vi "usrp get rx rates.vi"(8 "error in (no error)":errorcluster, 9 "rates_out":u64, 10 "chan":u64, 11 "h":u64) -> (0 "error out":errorcluster, 3 "function return":u32(ring))   [LabVIEW 2023, in "uhd.lvlib"]
doc: "UHD_API uhd_error uhd_usrp_get_rx_rates(\n uhd_usrp_handle h, size_t chan, uhd_meta_range_handle rates_out);"
uses:
  <userlib>/uhd/uhd.lvlib
  <userlib>/uhd/uhd.dll
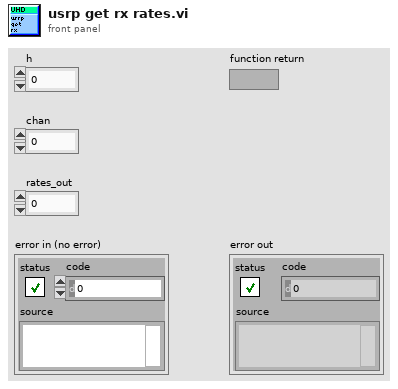
[diagram p1: front panel]
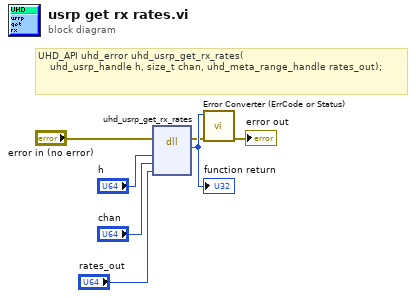
[diagram p0: block diagram]
diagram:
  # "UHD_API uhd_error uhd_usrp_get_rx_rates(\n    uhd_usrp_handle h, size_t chan, uhd_meta_range_handle rates_out);"
  n1 = dll-call lib="C:/Program Files/National Instruments/LabVIEW 2023/user.lib/uhd/uhd.*" fn="uhd_usrp_get_rx_rates"(error in="error in (no error)", "h"="h", "chan"="chan", "rates_out"="rates_out") -> (error out=w2:errorcluster, w7:u32)  [unwired: 5 in, 1 out]
  "function return" <- w7
  n2 = call <userlib>:"Error Converter (ErrCode or Status).vi"("error in (no error)"=w2, "error code"=w7) -> ("error out"=→"error out":errorcluster)  [unwired: 9 in]
